vi "Main.vi"(8 "error in (no error)":errorcluster, 11 "CascadeBase in":refnum<class "Cascade.lvclass">) -> (0 "error out":errorcluster, 3 "component":refnum<class "Cascade.lvclass">)   [LabVIEW 2012, in "Cascade.lvclass"]
doc: "Main VI of the component."
uses:
  Cascade.lvclass
  <vilib>/Distrio/Murmex/Murmex/command_enum.ctl
  Cascade.lvclass/Cascade.ctl
  <vilib>/Distrio/Murmex/InitialiseMessage/InitialiseMessage.lvclass
  <vilib>/Distrio/Murmex/GenericMessage/GenericMessage.lvclass
  <vilib>/Distrio/Murmex/TerminateMessage/TerminateMessage.lvclass
  <vilib>/Distrio/Murmex/ConfigureMessage/ConfigureMessage.lvclass
  <vilib>/Distrio/Murmex/StartMessage/run mode enum.ctl
  <vilib>/Distrio/Murmex/StopMessage/StopMessage.lvclass
  <vilib>/Distrio/Murmex/StartMessage/StartMessage.lvclass
  <vilib>/Distrio/Murmex/Murmex/update_cluster.ctl
  <vilib>/Distrio/Murmex/Murmex/Murmex.lvclass
  <vilib>/Distrio/Murmex/Murmex/Set configure at initialise.vi
  <vilib>/Distrio/Murmex/Murmex/Set log reference.vi
  <vilib>/Distrio/Murmex/Murmex/Set VI reference.vi
  <vilib>/Distrio/Murmex/Murmex/Get ID.vi
  <vilib>/Distrio/Murmex/Murmex/Set write log to disk.vi
  <vilib>/Distrio/Murmex/Message/Add or replace parameter.vi
  <vilib>/Distrio/Murmex/Message/Message.lvclass
panel:
  out "terminate?":bool
  in  "Tab Control":enum32{"Settings", "Phase comparison", "Debug"}(tab)
  out "Video":T1(plugin-control)
  in  "Exposure (ms)":u32
  in  "Gain":i16=3000
  in  "button:free run":bool
  out "Status":string
  in  "Reporting folder":path=path "C:/DATA"
  in  "Filename":string="trial"
  in  "save":bool
  in  "select ROIS":bool
  in  "PID gains":T2
  in  "button:quit":bool
  in  "button:configure":bool
  out "alignment":T1(plugin-control)
  out "good alignment?":bool
  out "translation":dbl[unit]
  out "pixel shift":dbl
  in  "send move":bool
  in  "AF":bool
  in  "set as focus":bool
  out "ROB":T1(plugin-control)
  out "ROY":T1(plugin-control)
  out "log":string
  in  "Component id":string="Cascade"
  in  "button:send command":bool
  in  "generic command":string
  in  "command":T3
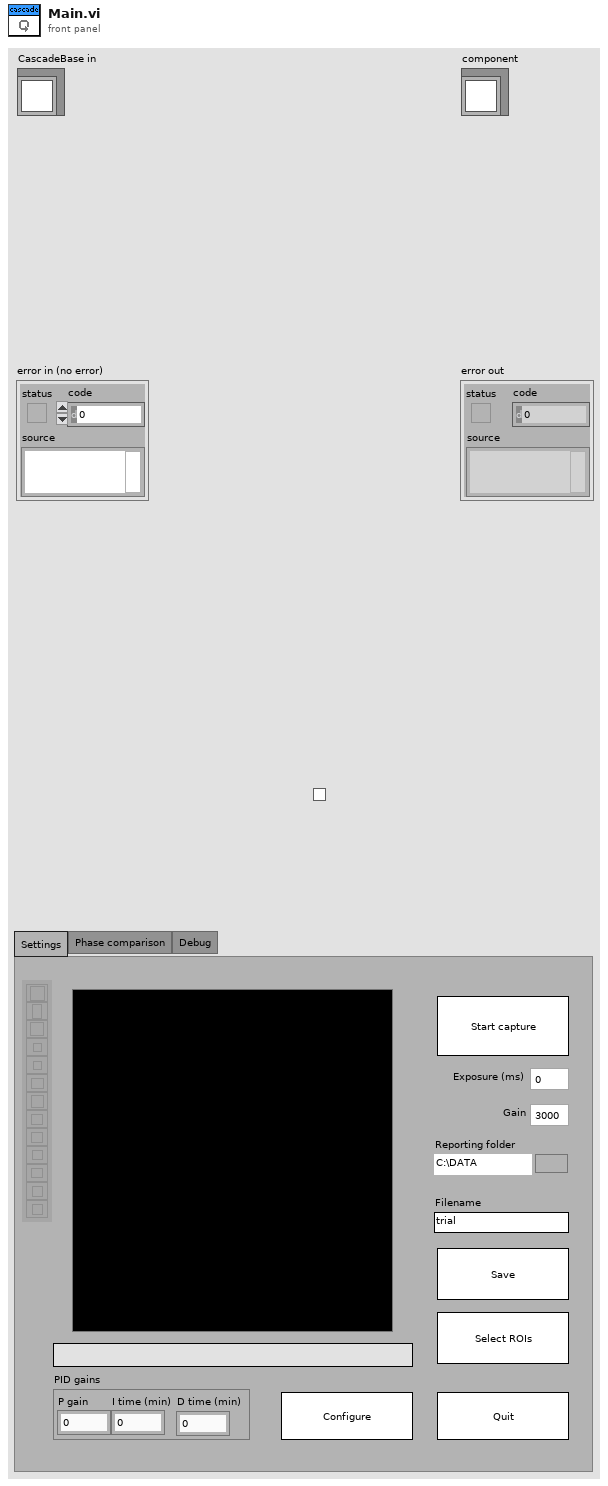
[diagram p1: front panel]
types:
  T1 = typedef "IMAQ Image.ctl" = refnum<image>
  T2 = cluster{"P gain":dbl, "I time (min)":dbl, "D time (min)":dbl}
  T3 = typedef "Murmex.lvlib/Murmex.lvclass/command_enum.ctl" = enum16{"null", "initialise", "reset", "terminate", "acknowledge", "update", "inspect", "inform", "proceed", "start", "stop", "fetch", "configure", "generic"}
  T4 = enum8{"Enabled", "Disabled", "Disabled and Grayed Out"}
  T5 = typedef "Murmex.lvlib/StartMessage.lvclass/run mode enum.ctl" = enum16{"infinite", "finite"}
  T6 = typedef "Murmex.lvlib/Murmex.lvclass/update_cluster.ctl" = cluster{"target ID":string, "key chains":string[], "values":variant[]}
  T7 = cluster{"proportional gain (Kc)":dbl, "integral time (Ti, min)":dbl, "derivative time (Td, min)":dbl}
  T8 = typedef "Murmex.lvclass/command_enum.ctl" = enum16{"null", "initialise", "reset", "terminate", "acknowledge", "update", "inspect", "inform", "proceed", "start", "stop", "fetch", "configure", "generic"}
  T9 = typedef "Murmex.lvclass/Event type enumerations.ctl" = enum16{"before", "after"}
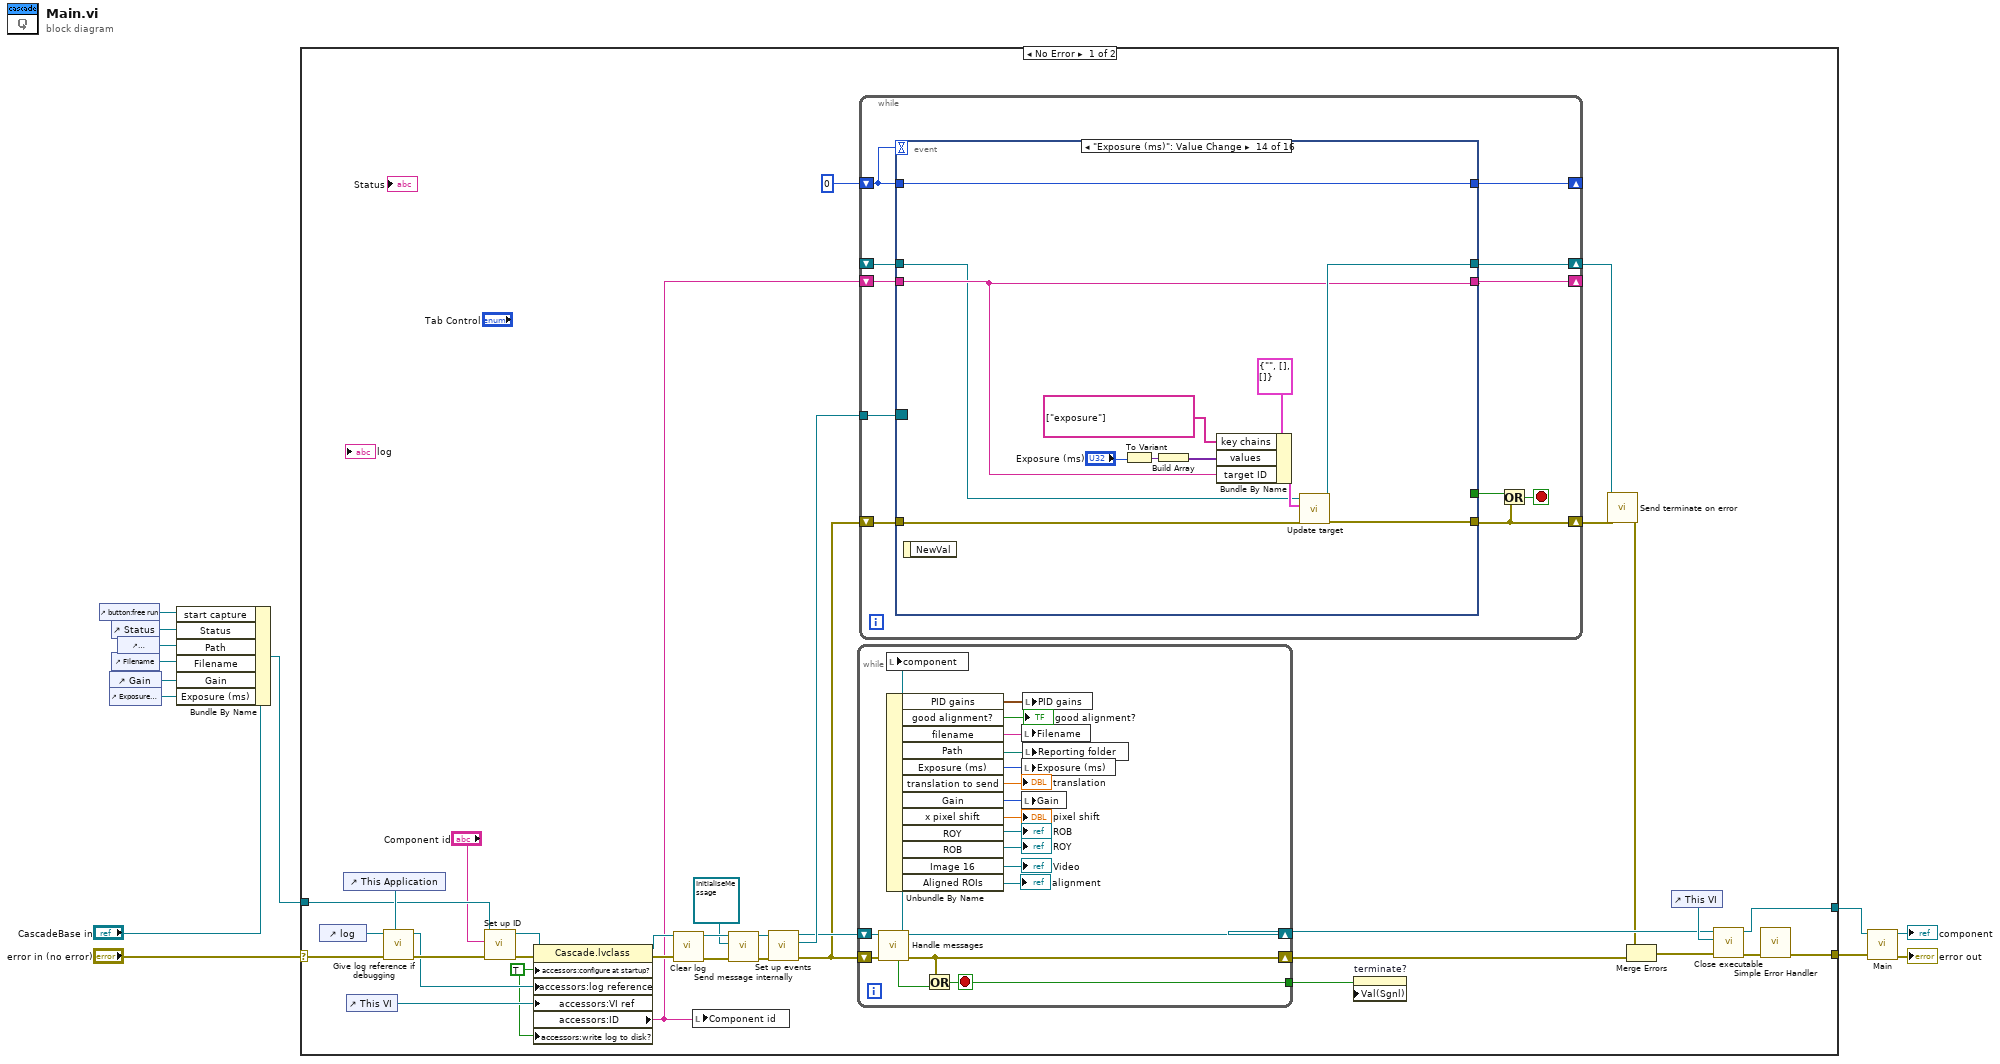
[diagram p0: block diagram]
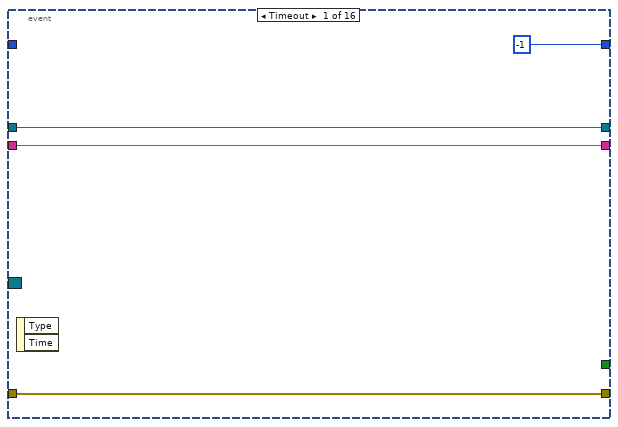
[diagram p2: hidden frame]
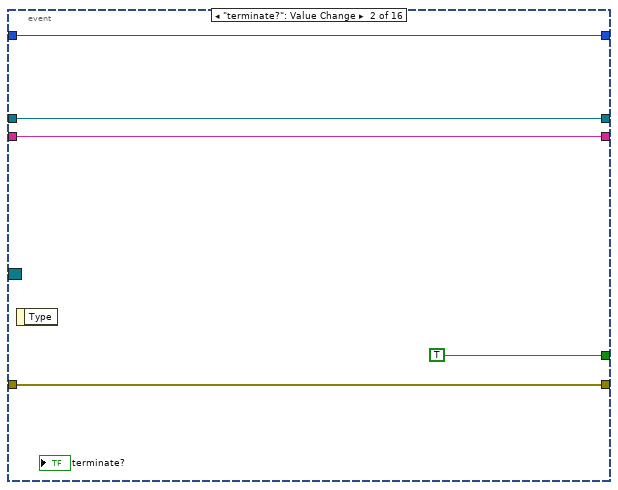
[diagram p3: hidden frame]
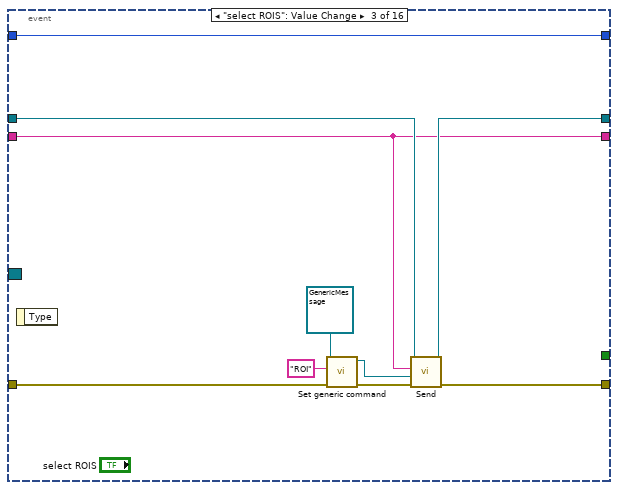
[diagram p4: hidden frame]
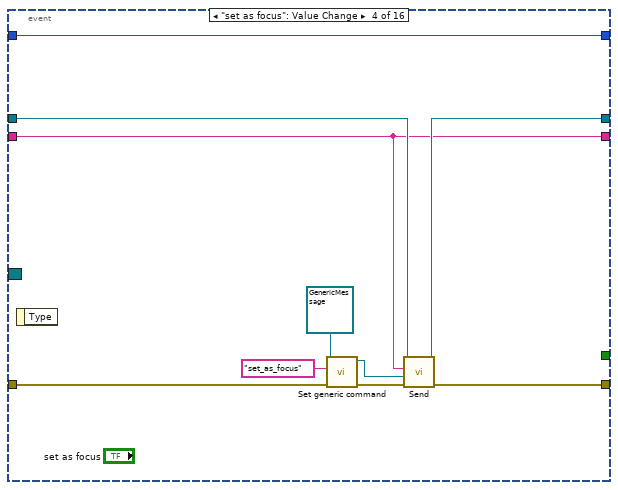
[diagram p5: hidden frame]
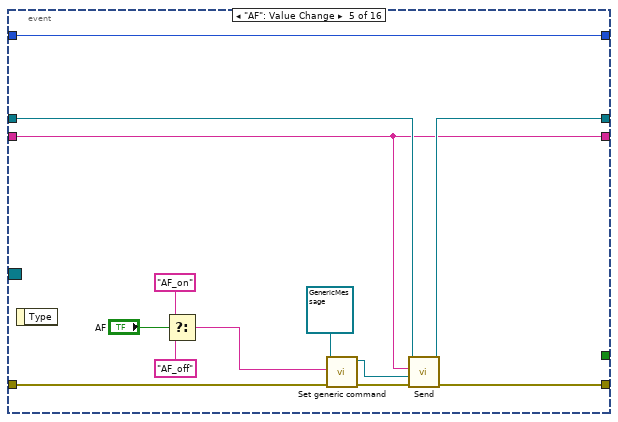
[diagram p6: hidden frame]
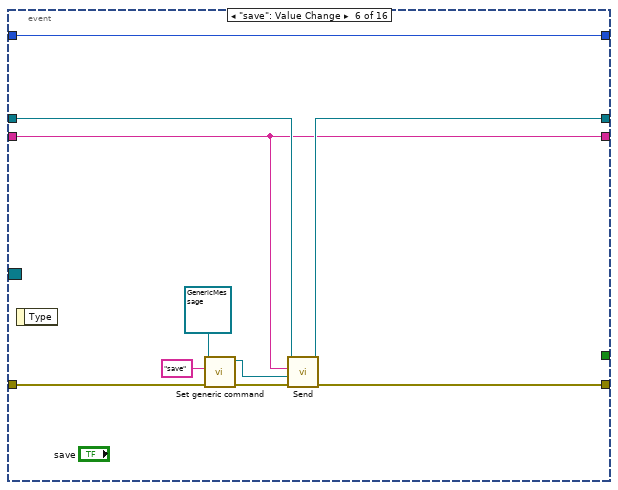
[diagram p7: hidden frame]
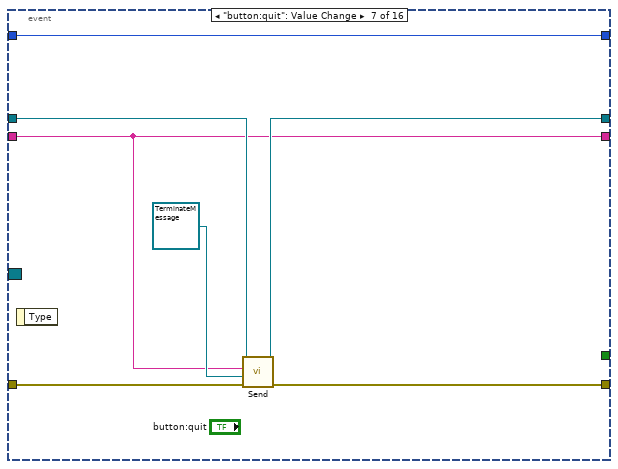
[diagram p8: hidden frame]
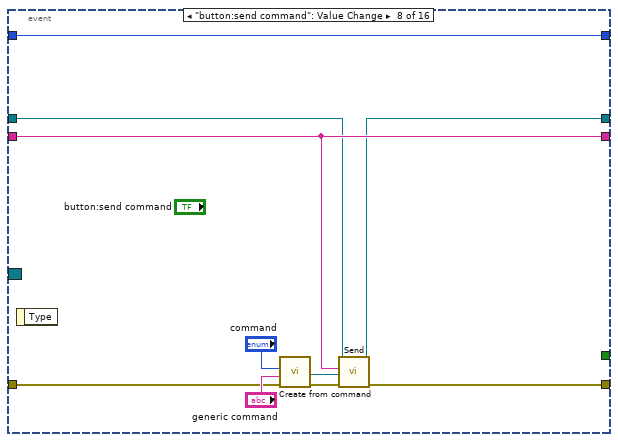
[diagram p9: hidden frame]
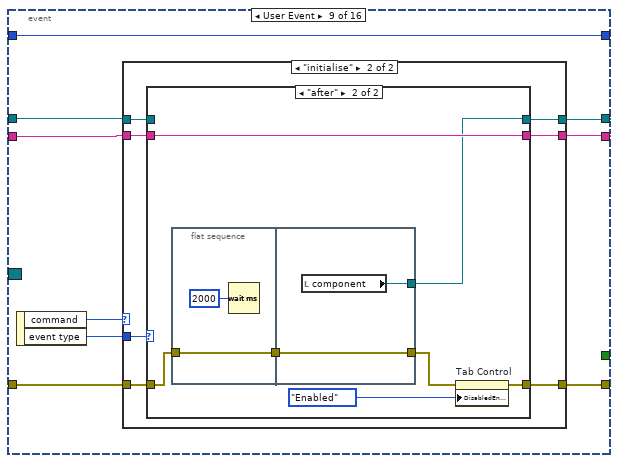
[diagram p10: hidden frame]
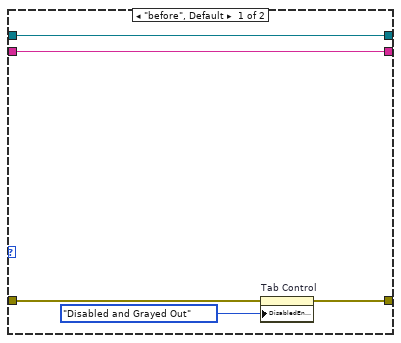
[diagram p12: hidden frame]
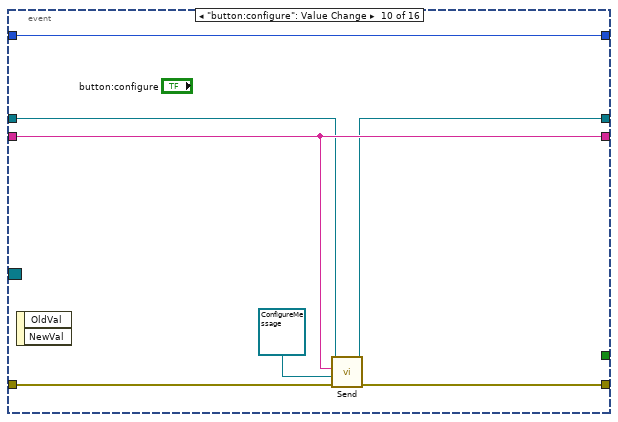
[diagram p13: hidden frame]
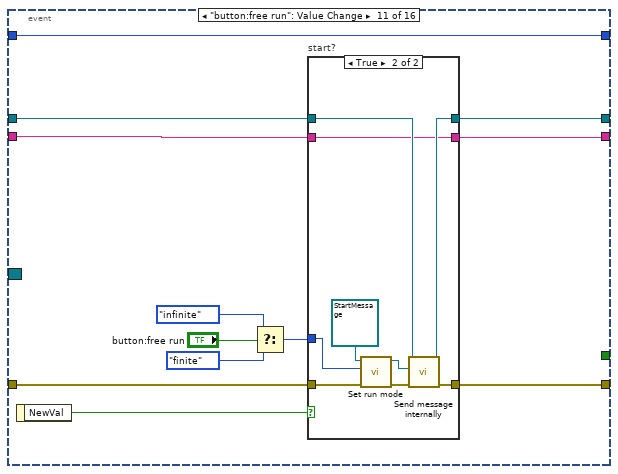
[diagram p14: hidden frame]
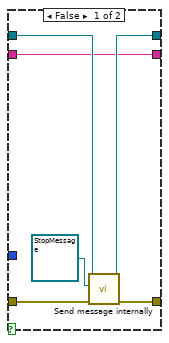
[diagram p15: hidden frame]
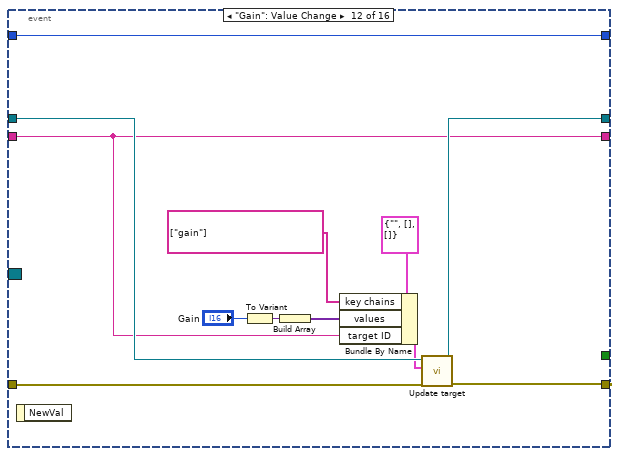
[diagram p16: hidden frame]
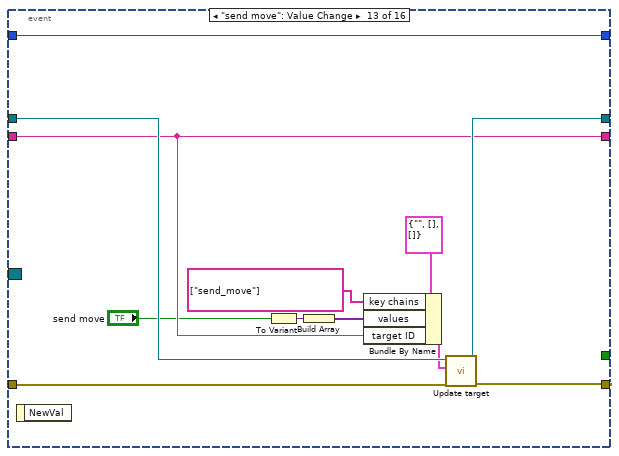
[diagram p17: hidden frame]
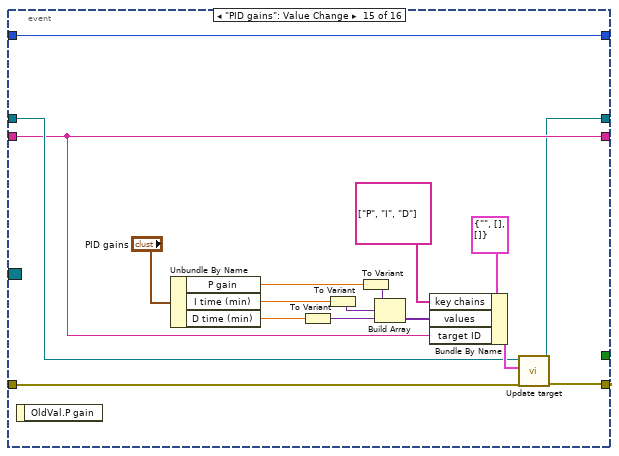
[diagram p18: hidden frame]
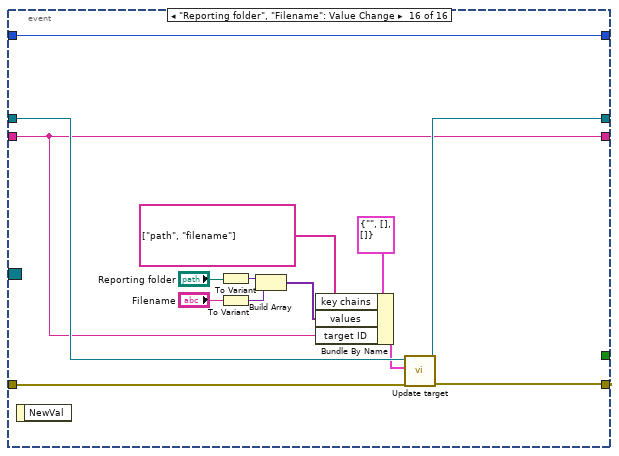
[diagram p19: hidden frame]
diagram:
  n1 = control-ref of="button:free run"() -> (w3:refnum<vi>)
  n2 = control-ref of="Gain"() -> (w1:refnum<vi>)
  n3 = control-ref of="Exposure (ms)"() -> (w2:refnum<vi>)
  n4 = control-ref of="Status"() -> (w4:refnum<vi>)
  n5 = control-ref of="Filename"() -> (w6:refnum<vi>)
  n6 = control-ref of="Reporting folder"() -> (w5:refnum<vi>)
  n7 = Bundle By Name(cluster="CascadeBase in", "start capture"=w3, "Status"=w4, "Path"=w5, "Filename"=w6, "Gain"=w1, "Exposure (ms)"=w2) -> (w10:refnum<class "Cascade.lvclass">)
  n8 = case shown="No Error" "error in (no error)" {
    selector: "error in (no error)" -> [w46 w283]
    tunnel: w10 -> [w45 w282]
    tunnel: [w19 w282] -> w9
    tunnel: [w17 w283] -> w7
    frame No Error {
      w15 = TRUE ("configure at startup?")
      n9 = control-ref of="log"() -> (w39:refnum<vi>)
      n10 = control-ref of="This Application"() -> (w47:refnum<vi>)
      n11 = control-ref of="This VI"() -> (w38:refnum<vi>)
      n12 = call "Give log reference if debugging.vi"("application ref"=w47, "error in (no error)"=w46, "log reference in"=w39) -> ("error out"=w44:errorcluster, "log reference out"=w40:refnum<vi>)  [unwired: 6 in, 1 out]
      n13 = call <vilib>:"Set up ID.vi"("error in (no error)"=w44, "component ID"="Component id", "MurmexBase in"=w45) -> ("error out"=w42:errorcluster, "MurmexBase out"=w41:refnum<class "Cascade.lvclass">)  [unwired: 6 in, 1 out]
      n14 = property class="Cascade.lvclass"(reference=w41, error in=w42, "accessors:configure at startup?"=w15, "accessors:log reference"=w40, "accessors:VI ref"=w38, "accessors:write log to disk?"=w15) -> (reference out=w31:refnum<class "Cascade.lvclass">, error out=w33:errorcluster, "accessors:ID"=w27:string)
      n15 = call <vilib>:"Clear log.vi"("error in (no error)"=w33, "MurmexBase in"=w31) -> ("error out"=w36:errorcluster, "MurmexBase out"=w37:refnum<class "Cascade.lvclass">)  [unwired: 8 in]
      n16 = local write "Component id"(w27) -> ()
      n17 = call <vilib>:"Send message internally.vi"("error in (no error)"=w36, "Message"=refnum<class "InitialiseMessage.lvclass"> refnum ("InitialiseMessage"), "Murmex in"=w37) -> ("error out"=w35:errorcluster, "Murmex out"=w34:refnum<class "Cascade.lvclass">)  [unwired: 7 in]
      n18 = call <vilib>:"Set up events.vi"("error in (no error)"=w35, "MurmexBase in"=w34) -> ("error out"=w28:errorcluster, "Event Registration Refnum"=w30:refnum<event-registration>, "MurmexBase out"=w29:refnum<class "Cascade.lvclass">)  [unwired: 7 in]
      n19 = while {
        shift-right: [w279] -> w14
        shift-left: w28 -> [w281]
        shift-right: [w276] -> w20
        shift-left: w29 -> [w277]
        tunnel: [w278] -> w16
        stop <- w278 stop-if-true
        n20 = call <vilib>:"Handle messages.vi"("error in (no error)"=w281, "Murmex in"=w277) -> ("error out"=w279:errorcluster, "Murmex out"=w276:refnum<class "Cascade.lvclass">, "terminated?"=w280:bool)  [unwired: 7 in]
        n21 = local write "component"(w276) -> ()
        n22 = Unbundle By Name(w276) -> ("PID gains"=w265:T7, "good alignment?"=→"good alignment?":bool, "filename"=w268:string, "Path"=w267:path, "Exposure (ms)"=w269:u32, "translation to send"=→"translation":dbl[unit], "Gain"=w270:i16, "x pixel shift"=→"pixel shift":dbl, "ROY"=→"ROY":T1, "ROB"=→"ROB":T1, "Image 16"=→"Video":T1, "Aligned ROIs"=→"alignment":T1)
        n23 = Or(x=w279, y=w280) -> (x .or. y?=w278:bool)
        n24 = local write "Filename"(w268) -> ()
        n25 = local write "Exposure (ms)"(w269) -> ()
        n26 = local write "Gain"(w270) -> ()
        n27 = local write "PID gains"(w265) -> ()
        n28 = local write "Reporting folder"(w267) -> ()
      }
      n29 = while {
        tunnel: w30 -> [w58]
        shift-right: [w50] -> w25
        shift-left: w28 -> [w57]
        shift-right: [w55] -> _
        shift-left: 0 -> [w54]
        shift-right: [w53] -> _
        shift-left: w27 -> [w56]
        shift-right: [w52] -> w24
        shift-left: _ -> [w51]
        stop <- w49 stop-if-true
        n30 = event shown="[13] \"Exposure (ms)\": Value Change" {
          selector: w58 -> [_ _ _ _ _ _ _ _ _ _ _ _ _ _ _ _]
          dyn-events: _ -> [_ _ _ _ _ _ _ _ _ _ _ _ _ _ _ _]
          timeout: w54 -> [_ _ _ _ _ _ _ _ _ _ _ _ _ _ _ _]
          tunnel: w57 -> [w61 w66 w73 w83 w97 w105 w117 w123 w136 w167 w180 w207 w219 w231 w242 w262]
          tunnel: w56 -> [w60 w65 w70 w80 w94 w101 w112 w121 w132 w165 w173 w197 w210 w223 w243 w253]
          tunnel: w54 -> [_ w63 w68 w78 w92 w110 w111 w118 w128 w169 w181 w199 w211 w224 w239 w254]
          tunnel: [-1 w63 w68 w78 w92 w110 w111 w118 w128 w169 w181 w199 w211 w224 w239 w254] -> w55
          tunnel: [w61 w66 w69 w79 w93 w104 w116 w122 w135 w166 w179 w208 w220 w232 w241 w263] -> w50
          tunnel: [w60 w65 w70 w80 w94 w101 w112 w121 w131 w165 w170 w197 w210 w223 w243 w253] -> w53
          tunnel: [w59 w64 w71 w81 w95 w102 w113 w119 w130 w163 w171 w206 w218 w230 w240 w261] -> w52
          tunnel: w51 -> [w59 w64 w72 w82 w96 w103 w114 w120 w129 w164 w172 w205 w217 w222 w244 w260]
          tunnel: [_ TRUE _ _ _ _ _ _ _ _ _ _ _ _ _ _] -> w48
          event Timeout {
            n31 = event-data() -> ()  [unwired: 1 in, 2 out]
          }
          event "terminate?": Value Change {
            n32 = event-data() -> ()  [unwired: 1 in, 1 out]
          }
          event "select ROIS": Value Change {
            n33 = event-data() -> ()  [unwired: 1 in, 1 out]
            n34 = call <vilib>:"Set generic command.vi"("error in (no error)"=w73, "generic command"="ROI", "GenericMessage in"=refnum<class "GenericMessage.lvclass"> refnum ("Message in")) -> ("error out"=w74:errorcluster, "GenericMessage out"=w76:refnum<class "GenericMessage.lvclass">)  [unwired: 7 in]
            n35 = call <vilib>:"Send.vi"("error in (no error)"=w74, "Message"=w76, "recipient"=w70, "Murmex in"=w72) -> ("error out"=w69:errorcluster, "Murmex out"=w71:refnum<class "Murmex.lvclass">)  [unwired: 6 in]
          }
          event "set as focus": Value Change {
            n36 = event-data() -> ()  [unwired: 1 in, 1 out]
            n37 = call <vilib>:"Set generic command.vi"("error in (no error)"=w83, "generic command"="set_as_focus", "GenericMessage in"=refnum<class "GenericMessage.lvclass"> refnum ("Message in")) -> ("error out"=w84:errorcluster, "GenericMessage out"=w86:refnum<class "GenericMessage.lvclass">)  [unwired: 7 in]
            n38 = call <vilib>:"Send.vi"("error in (no error)"=w84, "Message"=w86, "recipient"=w80, "Murmex in"=w82) -> ("error out"=w79:errorcluster, "Murmex out"=w81:refnum<class "Murmex.lvclass">)  [unwired: 6 in]
          }
          event "AF": Value Change {
            n39 = event-data() -> ()  [unwired: 1 in, 1 out]
            n40 = Select(t="AF_on" ("generic command"), s="AF", f="AF_off" ("generic command")) -> (s? t:f=w88:string)
            n41 = call <vilib>:"Set generic command.vi"("error in (no error)"=w97, "generic command"=w88, "GenericMessage in"=refnum<class "GenericMessage.lvclass"> refnum ("Message in")) -> ("error out"=w98:errorcluster, "GenericMessage out"=w100:refnum<class "GenericMessage.lvclass">)  [unwired: 7 in]
            n42 = call <vilib>:"Send.vi"("error in (no error)"=w98, "Message"=w100, "recipient"=w94, "Murmex in"=w96) -> ("error out"=w93:errorcluster, "Murmex out"=w95:refnum<class "Murmex.lvclass">)  [unwired: 6 in]
          }
          event "save": Value Change {
            n43 = event-data() -> ()  [unwired: 1 in, 1 out]
            n44 = call <vilib>:"Set generic command.vi"("error in (no error)"=w105, "generic command"="save", "GenericMessage in"=refnum<class "GenericMessage.lvclass"> refnum ("Message in")) -> ("error out"=w106:errorcluster, "GenericMessage out"=w108:refnum<class "GenericMessage.lvclass">)  [unwired: 7 in]
            n45 = call <vilib>:"Send.vi"("error in (no error)"=w106, "Message"=w108, "recipient"=w101, "Murmex in"=w103) -> ("error out"=w104:errorcluster, "Murmex out"=w102:refnum<class "Murmex.lvclass">)  [unwired: 6 in]
          }
          event "button:quit": Value Change {
            n46 = event-data() -> ()  [unwired: 1 in, 1 out]
            n47 = call <vilib>:"Send.vi"("error in (no error)"=w117, "Message"=refnum<class "TerminateMessage.lvclass"> refnum ("TerminateMessage"), "recipient"=w112, "Murmex in"=w114) -> ("error out"=w116:errorcluster, "Murmex out"=w113:refnum<class "Murmex.lvclass">)  [unwired: 6 in]
          }
          event "button:send command": Value Change {
            n48 = event-data() -> ()  [unwired: 1 in, 1 out]
            n49 = call <vilib>:"Create from command.vi"("error in (no error)"=w123, "generic command"="generic command", "command"="command") -> ("error out"=w124:errorcluster, "Message out"=w127:refnum<class "Message.lvclass">)  [unwired: 7 in]
            n50 = call <vilib>:"Send.vi"("error in (no error)"=w124, "Message"=w127, "recipient"=w121, "Murmex in"=w120) -> ("error out"=w122:errorcluster, "Murmex out"=w119:refnum<class "Murmex.lvclass">)  [unwired: 6 in]
          }
          event User Event {
            n51 = event-data() -> ("command"=w133:T8, "event type"=w134:T9)  [unwired: 1 in]
            n52 = case shown="\"initialise\"" w133 {
              tunnel: w134 -> [_ w146]
              tunnel: w136 -> [w137 w145]
              tunnel: w132 -> [w138 w144]
              tunnel: [w138 w143] -> w131
              tunnel: [w139 w142] -> w130
              tunnel: w129 -> [w139 w141]
              tunnel: [w137 w140] -> w135
              frame "null", Default {
              }
              frame "initialise" {
                n53 = case shown="\"after\"" w146 {
                  tunnel: w145 -> [w148 w153]
                  tunnel: [w147 w157] -> w140
                  tunnel: [w150 w156] -> w143
                  tunnel: w144 -> [w150 w156]
                  tunnel: [w151 w155] -> w142
                  tunnel: w141 -> [w151 _]
                  frame "before", Default {
                    n54 = property on="Tab Control" class="TabCtl (strict)"(error in=w148, "DisabledEnum"=T4."Disabled and Grayed Out" ("Disabled")) -> (error out=w147:errorcluster)  [unwired: 1 in, 1 out]
                  }
                  frame "after" {
                    n55 = flat-sequence {
                      tunnel: [w160] -> w154
                      tunnel: w153 -> [w160]
                      tunnel: [w162] -> w155
                      tunnel: [w161] -> w152
                      tunnel: w154 -> [w161]
                      frame #0 {
                        n56 = Wait (ms)(milliseconds to wait=u32 2000) -> ()  [unwired: 1 out]
                      }
                      frame #1 {
                        n57 = local read "component"() -> (w162:refnum<class "Cascade.lvclass">)
                      }
                    }
                    n58 = property on="Tab Control" class="TabCtl (strict)"(error in=w152, "DisabledEnum"=T4."Enabled" ("Disabled")) -> (error out=w157:errorcluster)  [unwired: 1 in, 1 out]
                  }
                }
              }
            }
          }
          event "button:configure": Value Change {
            n59 = event-data() -> ()  [unwired: 1 in, 2 out]
            n60 = call <vilib>:"Send.vi"("error in (no error)"=w167, "Message"=refnum<class "ConfigureMessage.lvclass"> refnum ("ConfigureMessage"), "recipient"=w165, "Murmex in"=w164) -> ("error out"=w166:errorcluster, "Murmex out"=w163:refnum<class "Murmex.lvclass">)  [unwired: 6 in]
          }
          event "button:free run": Value Change {
            n61 = event-data() -> ("NewVal"=w178:bool)  [unwired: 1 in]
            n62 = Select(t=run_mode_enum."infinite" ("run mode"), s="button:free run", f=run_mode_enum."finite" ("run mode")) -> (s? t:f=w174:T5)
            n63 = case "start?" shown="True" w178 {
              tunnel: w180 -> [w187 w191]
              tunnel: [w186 w194] -> w179
              tunnel: w172 -> [w185 w196]
              tunnel: [w184 w195] -> w171
              tunnel: w173 -> [w183 w193]
              tunnel: [w183 w193] -> w170
              tunnel: w174 -> [_ w192]
              frame False {
                n64 = call <vilib>:"Send message internally.vi"("error in (no error)"=w187, "Message"=refnum<class "StopMessage.lvclass"> refnum ("Distrio Murmex 1.5:StopMessage"), "Murmex in"=w185) -> ("error out"=w186:errorcluster, "Murmex out"=w184:refnum<class "Murmex.lvclass">)  [unwired: 7 in]
              }
              frame True {
                n65 = call <vilib>:"Set run mode.vi"("error in (no error)"=w191, "run mode"=w192, "StartMessage in"=refnum<class "StartMessage.lvclass"> refnum ("Message in")) -> ("error out"=w190:errorcluster, "StartMessage out"=w188:refnum<class "StartMessage.lvclass">)  [unwired: 7 in]
                n66 = call <vilib>:"Send message internally.vi"("error in (no error)"=w190, "Message"=w188, "Murmex in"=w196) -> ("error out"=w194:errorcluster, "Murmex out"=w195:refnum<class "Murmex.lvclass">)  [unwired: 7 in]
              }
            }
          }
          event "Gain": Value Change {
            n67 = event-data() -> ()  [unwired: 1 in, 1 out]
            n68 = To Variant(anything="Gain") -> (Variant=w203:variant)
            n69 = Build Array(w203) -> (w204:variant[])
            n70 = Bundle By Name(cluster=T6 {"target ID"="", "key chains"=[], "values"=[]} ("update cluster"), "key chains"=string[] ["gain"], "values"=w204, "target ID"=w197) -> (w201:T6)
            n71 = call <vilib>:"Update target.vi"("error in (no error)"=w207, "update cluster"=w201, "MurmexBase in"=w205) -> ("error out"=w208:errorcluster, "MurmexBase out"=w206:refnum<class "Murmex.lvclass">)  [unwired: 7 in]
          }
          event "send move": Value Change {
            n72 = event-data() -> ()  [unwired: 1 in, 1 out]
            n73 = To Variant(anything="send move") -> (Variant=w215:variant)
            n74 = Build Array(w215) -> (w216:variant[])
            n75 = Bundle By Name(cluster=T6 {"target ID"="", "key chains"=[], "values"=[]} ("update cluster"), "key chains"=string[] ["send_move"], "values"=w216, "target ID"=w210) -> (w213:T6)
            n76 = call <vilib>:"Update target.vi"("error in (no error)"=w219, "update cluster"=w213, "MurmexBase in"=w217) -> ("error out"=w220:errorcluster, "MurmexBase out"=w218:refnum<class "Murmex.lvclass">)  [unwired: 7 in]
          }
          event "Exposure (ms)": Value Change {
            n77 = event-data() -> ()  [unwired: 1 in, 1 out]
            n78 = To Variant(anything="Exposure (ms)") -> (Variant=w228:variant)
            n79 = Build Array(w228) -> (w229:variant[])
            n80 = Bundle By Name(cluster=T6 {"target ID"="", "key chains"=[], "values"=[]} ("update cluster"), "key chains"=string[] ["exposure"], "values"=w229, "target ID"=w223) -> (w226:T6)
            n81 = call <vilib>:"Update target.vi"("error in (no error)"=w231, "update cluster"=w226, "MurmexBase in"=w222) -> ("error out"=w232:errorcluster, "MurmexBase out"=w230:refnum<class "Murmex.lvclass">)  [unwired: 7 in]
          }
          event "PID gains": Value Change {
            n82 = event-data() -> ()  [unwired: 1 in, 1 out]
            n83 = Unbundle By Name("PID gains") -> ("P gain"=w237:dbl, "I time (min)"=w236:dbl, "D time (min)"=w235:dbl)
            n84 = To Variant(anything=w235) -> (Variant=w248:variant)
            n85 = To Variant(anything=w236) -> (Variant=w234:variant)
            n86 = To Variant(anything=w237) -> (Variant=w233:variant)
            n87 = Build Array(w233, w234, w248) -> (w249:variant[])
            n88 = Bundle By Name(cluster=T6 {"target ID"="", "key chains"=[], "values"=[]} ("update cluster"), "key chains"=string[] ["P", "I", "D"], "values"=w249, "target ID"=w243) -> (w246:T6)
            n89 = call <vilib>:"Update target.vi"("error in (no error)"=w242, "update cluster"=w246, "MurmexBase in"=w244) -> ("error out"=w241:errorcluster, "MurmexBase out"=w240:refnum<class "Murmex.lvclass">)  [unwired: 7 in]
          }
          event "Reporting folder", "Filename": Value Change {
            n90 = event-data() -> ()  [unwired: 1 in, 1 out]
            n91 = To Variant(anything="Reporting folder") -> (Variant=w258:variant)
            n92 = To Variant(anything="Filename") -> (Variant=w250:variant)
            n93 = Build Array(w258, w250) -> (w259:variant[])
            n94 = Bundle By Name(cluster=T6 {"target ID"="", "key chains"=[], "values"=[]} ("update cluster"), "key chains"=string[] ["path", "filename"], "values"=w259, "target ID"=w253) -> (w256:T6)
            n95 = call <vilib>:"Update target.vi"("error in (no error)"=w262, "update cluster"=w256, "MurmexBase in"=w260) -> ("error out"=w263:errorcluster, "MurmexBase out"=w261:refnum<class "Murmex.lvclass">)  [unwired: 7 in]
          }
        }
        n96 = Or(x=w48, y=w50) -> (x .or. y?=w49:bool)
      }
      n97 = property on="terminate?" class="Bool (strict)"("Val(Sgnl)"=w16) -> ()  [unwired: 2 in, 2 out]
      n98 = call <vilib>:"Send terminate on error.vi"("error in (no error)"=w25, "Murmex in"=w24) -> ("error out"=w18:errorcluster)  [unwired: 8 in, 1 out]
      n99 = Merge Errors(w18, w14) -> (w22:errorcluster)
      n100 = control-ref of="This VI"() -> (w21:refnum<vi>)
      n101 = call <vilib>:"Close executable.vi"("error in (no error)"=w22, "main VI ref (optional)"=w21, "MurmexBase in"=w20) -> ("error out"=w23:errorcluster, "MurmexBase out"=w19:refnum<class "Cascade.lvclass">)  [unwired: 7 in]
      n102 = call <vilib>:"Simple Error Handler.vi"("error in (no error)"=w23) -> ("error out"=w17:errorcluster)  [unwired: 4 in, 4 out]
    }
    frame Error {
    }
  }
  n103 = call-parent "Main.vi"("error in (no error)"=w7, "Murmex in"=w9) -> ("error out"=→"error out":errorcluster, "Murmex out"=→"component":refnum<class "Cascade.lvclass">)  [unwired: 8 in]
